vi "Actor Core.vi"(8 "error in":errorcluster, 11 "RDS Parent Actor in":refnum<class "RDS Parent Actor.lvclass">) -> (0 "error out":errorcluster, 3 "Actor out":refnum<class "Actor.lvclass">)   [LabVIEW 2015]
doc: "(<B>Filename</B>: Actor Framework.lvlib:Actor.lvclass:Actor Core.vi)\n\nReceives messages to the actor, reacts to them, and initiates any error handling that may shut the actor down.\n\nDescendant classes may override this VI to append parallel tasks for the actor to complete while it handles messages. Overrides use the Call Parent Method node."
uses:
  RDS Parent Actor.lvclass
  <vilib>/ActorFramework/Actor/Actor.lvclass
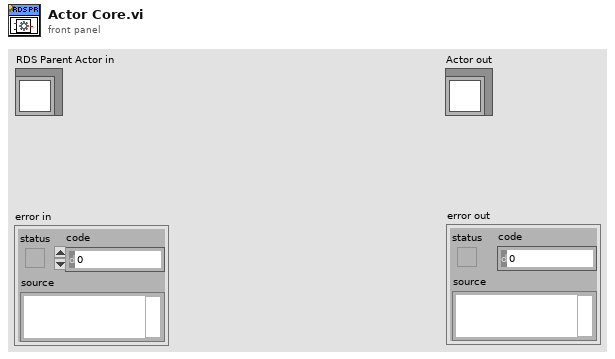
[diagram p1: front panel]
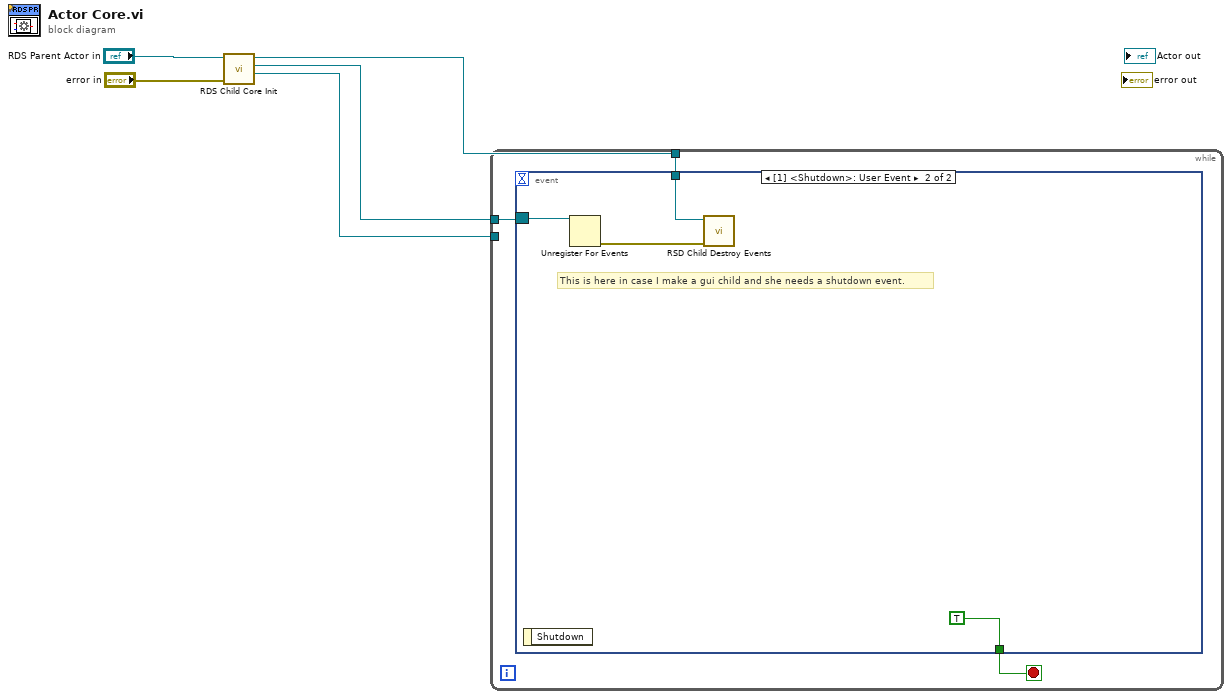
[diagram p0: block diagram]
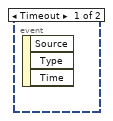
[diagram p2: hidden frame]
diagram:
  n1 = call "RDS Child Core Init.vi"("error in (no error)"="error in", "RDS Parent Actor in"="RDS Parent Actor in") -> ("error out"=w1:errorcluster, "RDS Router Enqeuer"=w5:refnum<class "Message Enqueuer.lvclass">, "Event Registration Refnum"=w3:refnum<event-registration>, "RDS Parent Actor out"=w4:refnum<class "RDS Parent Actor.lvclass">)  [unwired: 6 in]
  n2 = while {
    tunnel: w5 -> [_]
    tunnel: w4 -> [w10]
    tunnel: w3 -> [w9]
    stop <- w11 stop-if-true
    n3 = event shown="[1] <Shutdown>: User Event" {
      selector: w9 -> [_ w14]
      dyn-events: _ -> [_ _]
      timeout: _ -> [_ _]
      tunnel: [_ TRUE] -> w11
      tunnel: w10 -> [_ w13]
      event Timeout {
        n4 = event-data() -> ()  [unwired: 1 in, 3 out]
      }
      event User Event {
        # "This is here in case I make a gui child and she needs a shutdown event."
        n5 = event-data() -> ()  [unwired: 1 in, 1 out]
        n6 = Unregister For Events(event registration refnum=w14) -> (error out=w12:errorcluster)  [unwired: 1 in]
        n7 = call "RSD Child Destroy Events.vi"("error in (no error)"=w12, "RDS Parent Actor in"=w13) -> ()  [unwired: 8 in, 2 out]
      }
    }
  }
